vi "Create MsgList File.vi"(8 "error in (no error)":errorcluster, 11 "Function in":refnum<class "Function.lvclass">) -> (0 "error out":errorcluster, 3 "Function out":refnum<class "Function.lvclass">)   [LabVIEW 2016, in "Function Actor.lvlib" / "Function.lvclass"]
uses:
  <userlib>/Common Components/Function Actor/Function.lvclass
  <userlib>/Common Components/Function Actor/Function.lvclass/Function.ctl
  <userlib>/Common Components/Common/Common.lvlib
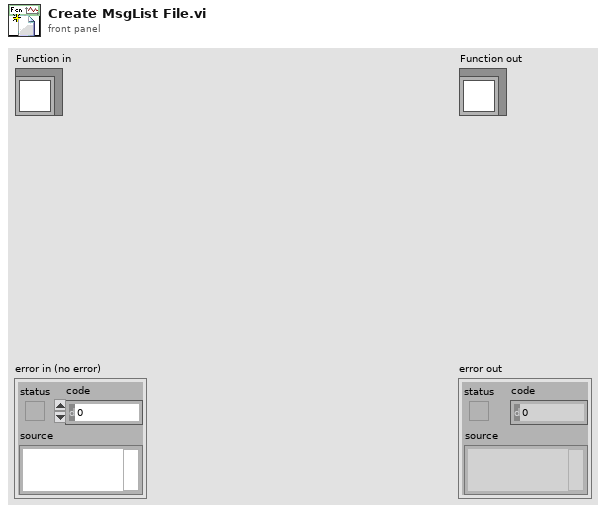
[diagram p1: front panel]
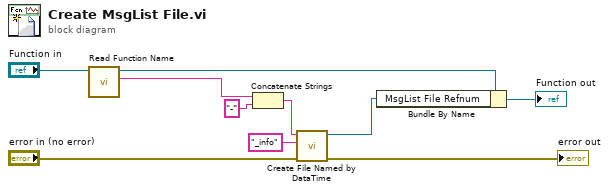
[diagram p0: block diagram]
diagram:
  n1 = call <userlib>:"Read Function Name.vi"("Function in"="Function in") -> ("Function Name"=w5:string, "Function out"=w9:refnum<class "Function.lvclass">)  [unwired: 8 in, 1 out]
  n2 = Concatenate Strings(w5, "-" ("string")) -> (w7:string)
  n3 = call <userlib>:"Create File Named by DataTime.vi"("error in (no error)"="error in (no error)", "suffix"="_info", "prefix"=w7) -> ("error out"=→"error out":errorcluster, "Byte Stream File out"=w3:refnum<file>)  [unwired: 7 in]
  n4 = Bundle By Name(cluster=w9, "MsgList File Refnum"=w3) -> (→"Function out":refnum<class "Function.lvclass">)
